vi "Judge Node Symbols.vi"(8 "error in (no error)":errorcluster, 10 "Tag":string, 11 "TreeControl in":refnum<vi>) -> (0 "error out":errorcluster, 2 "Selected?":bool, 3 "TreeControl out":refnum<vi>)   [LabVIEW 2023, in "DSLV_Tree.lvlib"]
uses:
  DSLV_Tree.lvlib
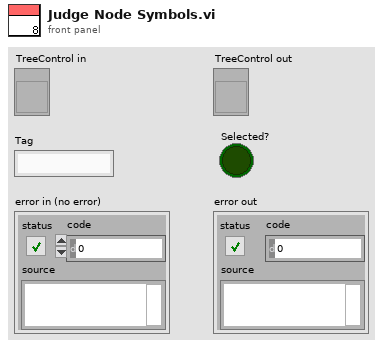
[diagram p1: front panel]
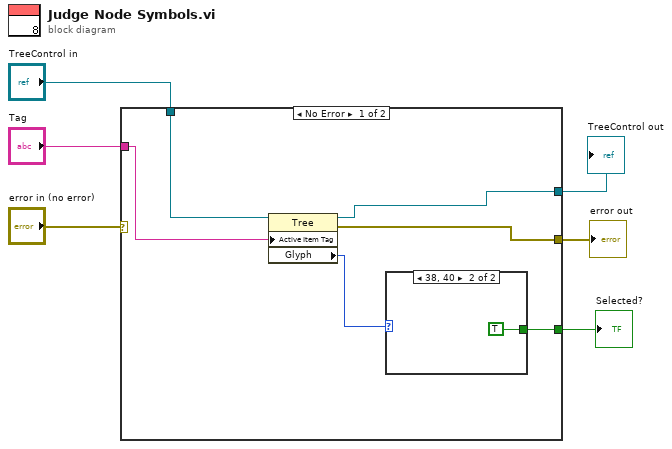
[diagram p0: block diagram]
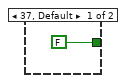
[diagram p2: hidden frame]
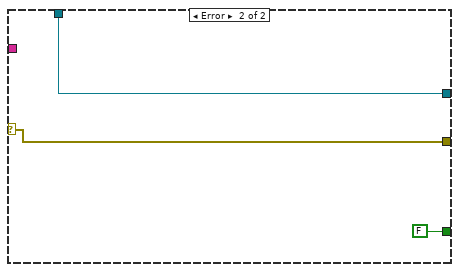
[diagram p3: hidden frame]
diagram:
  n1 = case shown="No Error" "error in (no error)" {
    selector: "error in (no error)" -> [_ w16]
    tunnel: [w12 w16] -> w6
    tunnel: [w11 w17] -> w5
    tunnel: "Tag" -> [w10 _]
    tunnel: "TreeControl in" -> [w9 w17]
    tunnel: [w7 FALSE] -> w1
    frame No Error {
      n2 = property on="Property Node" class="Tree"(reference=w9, "Active Item Tag"=w10) -> (reference out=w11:refnum<vi>, error out=w12:errorcluster, "Glyph"=w8:i32)  [unwired: 1 in]
      n3 = case shown="38, 40" w8 {
        tunnel: [FALSE TRUE] -> w7
        frame 37, Default {
        }
        frame 38, 40 {
        }
      }
    }
    frame Error {
    }
  }
  "error out" <- w6
  "TreeControl out" <- w5
  "Selected?" <- w1
